vi "controlOutput.vi"(7 "Set":bool, 8 "error in":errorcluster, 9 "enable output in":bool=TRUE, 10 "axis in":u8, 11 "connection ID":refnum<k5>) -> (0 "error out":errorcluster, 1 "enable output out":bool=TRUE, 2 "axis out":u8, 3 "connection ID":refnum<k5>)   [LabVIEW 2016, in "AMC_VIs.lvlib"]
doc: "This function retrieves or sets the status of the output relays of the selected axis."
uses:
  AMC_VIs.lvlib
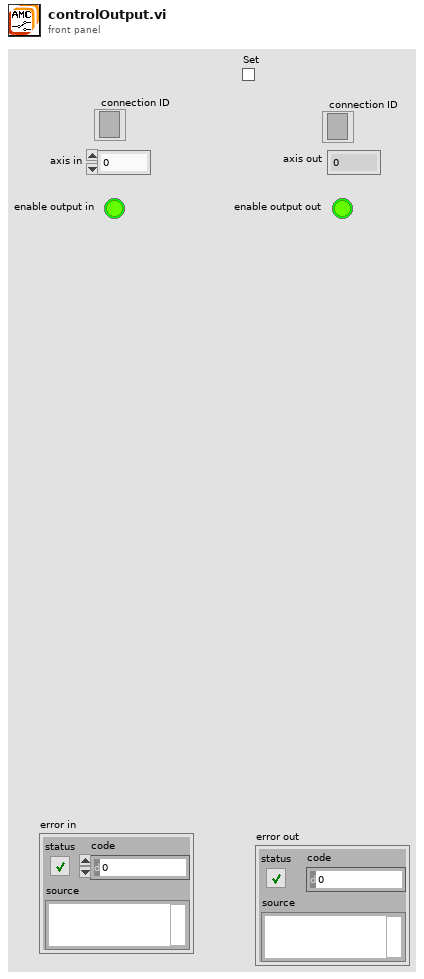
[diagram p1: front panel]
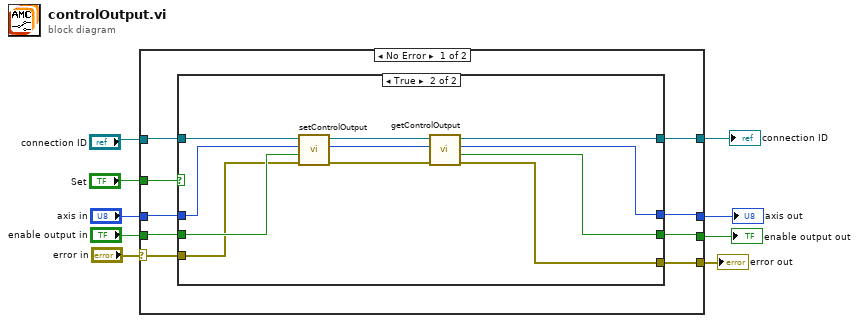
[diagram p0: block diagram]
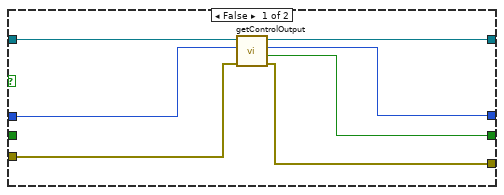
[diagram p2: hidden frame]
diagram:
  n1 = case shown="No Error" "error in" {
    selector: "error in" -> [w10 w40]
    tunnel: "axis in" -> [w16 w38]
    tunnel: [w11 w40] -> w1
    tunnel: [w15 w38] -> w8
    tunnel: "Set" -> [w12 _]
    tunnel: [w13 w39] -> w6
    tunnel: "enable output in" -> [w14 w39]
    tunnel: [w18 w37] -> w4
    tunnel: "connection ID" -> [w17 w37]
    frame No Error {
      n2 = case shown="True" w12 {
        tunnel: [w24 w32] -> w18
        tunnel: w17 -> [w25 w36]
        tunnel: w16 -> [w21 w29]
        tunnel: [w19 w27] -> w15
        tunnel: [w22 w26] -> w13
        tunnel: w14 -> [_ w35]
        tunnel: [w23 w28] -> w11
        tunnel: w10 -> [w20 w34]
        frame False {
          n3 = call "getControlOutput.vi"("error in"=w20, "axis"=w21, "connection ID"=w25) -> ("error out"=w23:errorcluster, "enabled"=w22:bool, "axis_out"=w19:i32, "connection ID"=w24:refnum<k5>)  [unwired: 5 in]
        }
        frame True {
          n4 = call "setControlOutput.vi"("error in"=w34, "enable"=w35, "axis"=w29, "connection ID"=w36) -> ("error out"=w31:errorcluster, "axis_out"=w30:i32, "connection ID"=w33:refnum<k5>)  [unwired: 5 in]
          n5 = call "getControlOutput.vi"("error in"=w31, "axis"=w30, "connection ID"=w33) -> ("error out"=w28:errorcluster, "enabled"=w26:bool, "axis_out"=w27:i32, "connection ID"=w32:refnum<k5>)  [unwired: 5 in]
        }
      }
    }
    frame Error {
    }
  }
  "error out" <- w1
  "axis out" <- w8
  "enable output out" <- w6
  "connection ID" <- w4
